vi "Pcre2JitMatch8.vi"(5 "pContext":u64 format="%.0x", 6 "pMatchData":u64 format="%.0x", 7 "Options":u32 format="%.0x", 8 "error in":errorcluster, 9 "StartOffset":u64, 10 "Subject":string, 11 "pCode":u64 format="%.0x") -> (0 "error out":errorcluster, 2 "MatchResult":i32, 3 "pCode":u64 format="%.0x", 4 "pMatchData":u64 format="%.0x")   [LabVIEW 2021, in "libpcre2-8.lvlib"]
uses:
  libpcre2-8.lvlib
  libpcre2-8-x32.dll
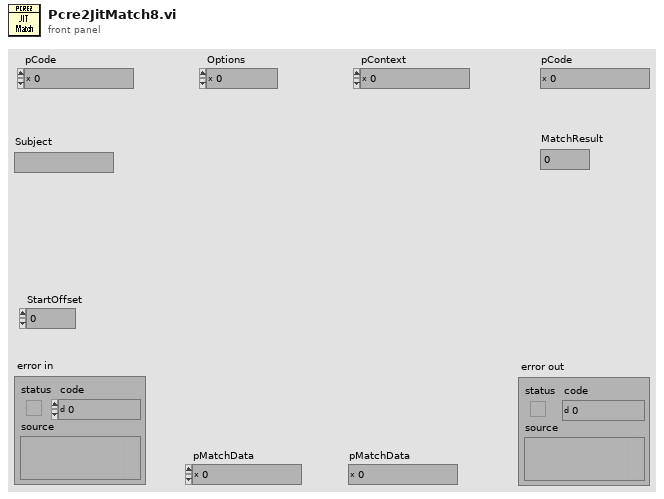
[diagram p1: front panel]
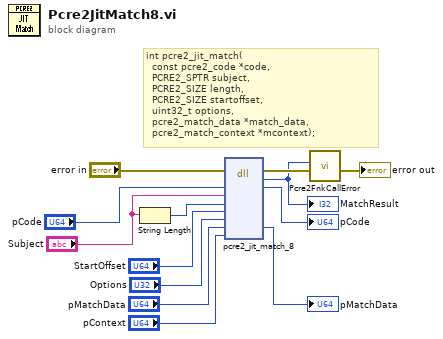
[diagram p0: block diagram]
diagram:
  # "int pcre2_jit_match(\n  const pcre2_code *code, \n  PCRE2_SPTR subject, \n  PCRE2_SIZE length, \n  PCRE2_SIZE startoffset, \n  uint32_t options, \n  pcre2_match_data *match_data, \n  pcre2_match_context *mcontext);"
  n1 = String Length(string="Subject") -> (length=w2:i32)
  n2 = dll-call lib="libpcre2-8-x*.dll" fn="pcre2_jit_match_8"(error in="error in", "code"="pCode", "subject"="Subject", "length"=w2, "startoffset"="StartOffset", "options"="Options", "match_data"="pMatchData", "mcontext"="pContext") -> (error out=w9:errorcluster, "result"=w3:i32, "code"=→"pCode":u64, "match_data"=→"pMatchData":u64)  [unwired: 7 in, 1 out]
  "MatchResult" <- w3
  n3 = call "Pcre2FnkCallError.vi"("error in"=w9, "ErrorCode"=w3) -> ("error out"=→"error out":errorcluster)  [unwired: 9 in]
